vi "RegisterconvertArrayLV86.vi"(1 "LittleEndian? (F)":bool, 2 "Register Array":u16[](array[numeric])) -> (0 "Converted Array":sgl[](array[numeric]))   [LabVIEW 2014]
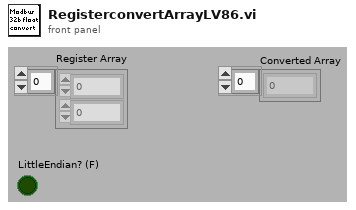
[diagram p1: front panel]
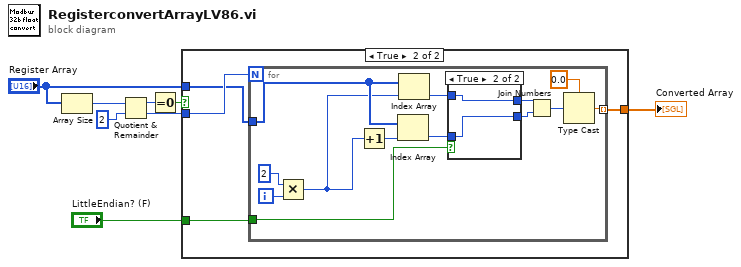
[diagram p0: block diagram]
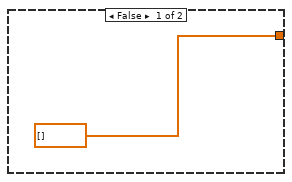
[diagram p2: hidden frame]
diagram:
  n1 = Array Size(array="Register Array") -> (size(s)=w8:i32)
  n2 = Quotient & Remainder(x=w8, y=2) -> (x-y*floor(x/y)=w6:i32, floor(x/y)=w3:i32)
  n3 = Equal To 0?(x=w6) -> (x = 0?=w5:bool)
  n4 = case shown="True" w5 {
    tunnel: "Register Array" -> [_ w12]
    tunnel: w3 -> [_ w13]
    tunnel: [sgl[] [] w11] -> w2
    tunnel: "LittleEndian? (F)" -> [_ w10]
    frame False {
    }
    frame True {
      n5 = for {
        N: w13 -> [_]
        tunnel: w12 -> [w16]
        tunnel: [w22] -> w11 mode=indexing
        tunnel: w10 -> [w17]
        i -> [w26]
        n6 = Multiply(x=2, y=w26) -> (x*y=w14:i32)
        n7 = Increment(x=w14) -> (x+1=w15:i32)
        n8 = Index Array(array=w16, index=w15) -> (element=w21:u16)
        n9 = Index Array(array=w16, index=w14) -> (element=w20:u16)
        n10 = case shown="True" w17 {
          tunnel: [w28 w30] -> w19
          tunnel: w21 -> [w27 w30]
          tunnel: [w27 w29] -> w18
          tunnel: w20 -> [w28 w29]
          frame False {
          }
          frame True {
          }
        }
        n11 = Join Numbers(hi=w18, lo=w19) -> ((hi.lo)=w24:u32)
        n12 = Type Cast(type=sgl 0.0, x=w24) -> (*(type *) &x=w22:sgl)
      }
    }
  }
  "Converted Array" <- w2
